vi "rvc Invert Matrix.vi"(11 "output":dbl) -> (3 "Inverse Matrix":T1)   [LabVIEW 2013]
uses:
  <vilib>/Analysis/Matrix/Datatypes/RealMatrix.ctl
  <vilib>/Analysis/baseanly.llb/Real Inverse Matrix.vi
  <vilib>/imath/engines/lvmath2/RunTimeEngine/BuiltInFunctions/inv/NIMS_inv(GM).vi
  <vilib>/imath/engines/lvmath2/RunTimeEngine/ErrorHandling/NIMS_Error From Error Code.vi
  <vilib>/imath/engines/lvmath2/RunTimeEngine/NodeEndStatement/NIMS_NodeEndStatement_Output.vi
  <vilib>/imath/engines/lvmath2/RunTimeEngine/ErrorHandling/NIMS_Finalize Error.vi
  <vilib>/Analysis/NI_AALBase.lvlib
  <vilib>/Analysis/Matrix/NI_Matrix.lvlib
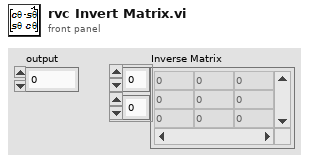
[diagram p1: front panel]
types:
  T1 = typedef "NI_Matrix.lvlib/RealMatrix.ctl" = dbl[][]
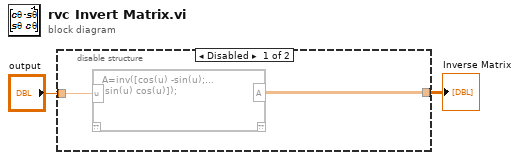
[diagram p0: block diagram]
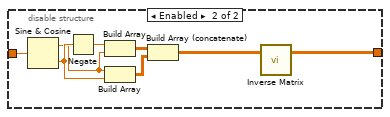
[diagram p2: hidden frame]
diagram:
  n1 = disable-structure "Diagram Disable Structure" shown="Disabled" {
    disable-tunnel: [w4 w41] -> w1
    disable-tunnel: "output" -> [w3 w44]
    frame Disabled {
      n2 = mathscript code="A=inv([cos(u) -sin(u);...\n sin(u) cos(u)]);"("u"=w3) -> ("A"=w4:dbl[][])  [unwired: 1 in, 1 out]
    }
    frame Enabled {
      n3 = Sine & Cosine(0:w44) -> (1:w43:dbl, 2:w45:dbl)
      n4 = Negate(x=w45) -> (-x=w46:dbl)
      n5 = Build Array ("Build Matrix 2")(w46, w43) -> (w48:T1)
      n6 = Build Array ("Build Matrix")(w43, w45) -> (w47:T1)
      n7 = Build Array (concatenate) ("Build Matrix 3")(w48, w47) -> (w42:T1)
      n8 = call-poly <vilib>:"Inverse Matrix.vi"("Input Matrix"=w42) -> ("Inverse Matrix"=w41:T1)  [unwired: 1 in, 1 out]
    }
  }
  "Inverse Matrix" <- w1
